vi "Enable-Disable ReaderFilter.vi"(8 "error in (no error)":errorcluster, 9 "Enable/Disable":bool, 10 "Baud Rate":u32=38400, 11 "COM Port":refnum<visa-resource-name>="COM4") -> (0 "error out":errorcluster, 1 "received str":string, 3 "Result":bool)   [LabVIEW 2018]
panel:
  # "Enable / Disable Reader Filter"
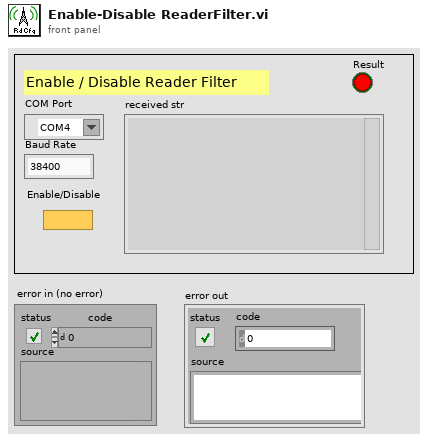
[diagram p1: front panel]
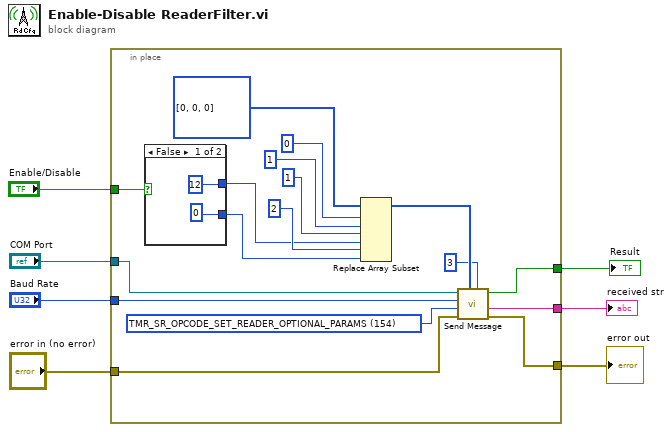
[diagram p0: block diagram]
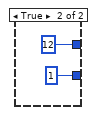
[diagram p2: hidden frame]
diagram:
  n1 = in-place {
    in-place-border: "Baud Rate" -> [w24]
    in-place-border: "COM Port" -> [w23]
    in-place-border: "error in (no error)" -> [w21]
    in-place-border: [w20] -> w4
    in-place-border: [w19] -> w3
    in-place-border: [w18] -> w2
    in-place-border: "Enable/Disable" -> [w11]
    w22 = u16 154 items=["TMR_SR_OPCODE_VERSION"=3, "TMR_SR_OPCODE_SET_BAUD_RATE"=6, "TMR_SR_OPCODE_READ_TAG_ID_SINGLE"=33, "TMR_SR_OPCODE_READ_TAG_ID_MULTIPLE"=34, "TMR_SR_OPCODE_WRITE_TAG_ID"=35, "TMR_SR_OPCODE_WRITE_TAG_DATA"=36, "TMR_SR_OPCODE_KILL_TAG"=38, "TMR_SR_OPCODE_READ_TAG_DATA"=40, "TMR_SR_OPCODE_CLEAR_TAG_ID_BUFFER"=42, "TMR_SR_OPCODE_MULTI_PROTOCOL_TAG_OP"=47, "TMR_SR_OPCODE_GET_READ_TX_POWER"=98, "TMR_SR_OPCODE_GET_WRITE_TX_POWER"=100, "TMR_SR_OPCODE_GET_POWER_MODE"=104, "TMR_SR_OPCODE_GET_READER_OPTIONAL_PARAMS"=106, "TMR_SR_OPCODE_GET_PROTOCOL_PARAM"=107, "TMR_SR_OPCODE_SET_ANTENNA_PORT"=145, "TMR_SR_OPCODE_SET_TAG_PROTOCOL"=147, "TMR_SR_OPCODE_SET_READ_TX_POWER"=146, "TMR_SR_OPCODE_SET_WRITE_TX_POWER"=148, "TMR_SR_OPCODE_SET_REGION"=151, "TMR_SR_OPCODE_SET_READER_OPTIONAL_PARAMS"=154, "TMR_SR_OPCODE_SET_PROTOCOL_PARAM"=155] ("Opcode Constant")
    n2 = case shown="False" w11 {
      tunnel: [u8 12 ("index") u8 12 ("index")] -> w10
      tunnel: [u8 0 ("index") u8 1 ("index")] -> w9
      frame False {
      }
      frame True {
      }
    }
    n3 = Replace Array Subset(array=u8[] [0, 0, 0], new element #1=1 ("index"), index #1=0 ("index"), new element #2=w10, index #2=1 ("index"), new element #3=w9, index #3=2 ("index")) -> (w16:u8[])
    n4 = call "Send Message.vi"("Size"=u8 3, "Data"=w16, "error in (no error)"=w21, "Opcode"=w22, "Baud Rate"=w24, "COM Port"=w23) -> ("error out"=w20:errorcluster, "received str"=w18:string, "Result"=w19:bool)  [unwired: 2 in, 1 out]
  }
  "error out" <- w4
  "Result" <- w3
  "received str" <- w2
